vi "Init B.vi"(8 "error in (no error)":errorcluster, 10 "Numeric":dbl, 11 "DA Child B in":refnum<class "DA Child B.lvclass">) -> (0 "error out":errorcluster, 3 "DA Child B out":refnum<class "DA Child B.lvclass">)   [LabVIEW 2020, in "Display As.lvlib" / "DA Child B.lvclass"]
uses:
  DA Child B.lvclass
  DA Child B.lvclass/DA Child B.ctl
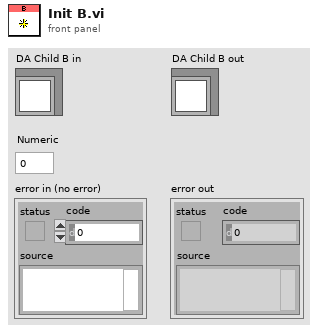
[diagram p1: front panel]
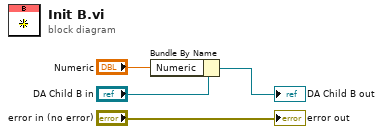
[diagram p0: block diagram]
diagram:
  n1 = Bundle By Name(cluster="DA Child B in", "Numeric"="Numeric") -> (→"DA Child B out":refnum<class "DA Child B.lvclass">)
  "error out" <- "error in (no error)"
